vi "FGV_Timer.vi"(7 "Timer action (read)":T1=enum."Run") -> (3 "Numeric":dbl)   [LabVIEW 2020]
uses:
  #typedef_FGV_TimerAction_ex_4.ctl
panel:
  out "Time Elapsed?":bool
  in  "TimeToElapse (s)":dbl=10.0
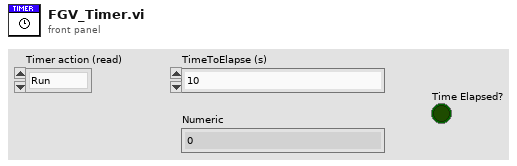
[diagram p1: front panel]
types:
  T1 = typedef "#typedef_FGV_TimerAction_ex_4.ctl" = enum16{"Reset", "Run", "Pause"}
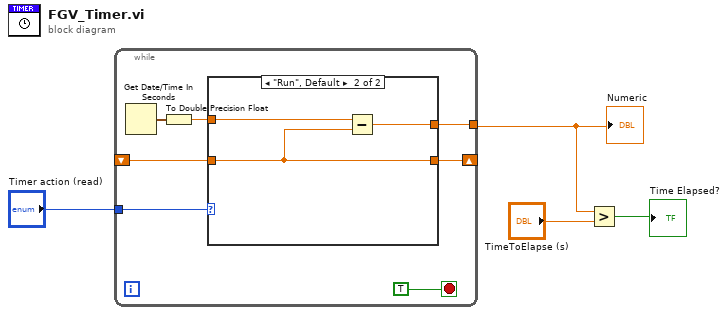
[diagram p0: block diagram]
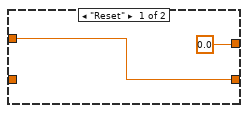
[diagram p2: hidden frame]
diagram:
  n1 = while {
    tunnel: "Timer action (read)" -> [w11]
    shift-right: [w8] -> _
    shift-left: _ -> [w6]
    tunnel: [w5] -> w3
    stop <- TRUE stop-if-true
    n2 = Get Date/Time In Seconds() -> (seconds since 1Jan1904=w9:timestamp)
    n3 = To Double Precision Float(number=w9) -> (double precision float=w7:dbl)
    n4 = case shown="\"Run\", Default" w11 {
      tunnel: [w13 w14] -> w8
      tunnel: w7 -> [w13 w16]
      tunnel: w6 -> [_ w14]
      tunnel: [0.0 w15] -> w5
      frame "Reset" {
      }
      frame "Run", Default {
        n5 = Subtract(x=w16, y=w14) -> (x-y=w15:dbl)
      }
    }
  }
  "Numeric" <- w3
  n6 = Greater?(x=w3, y="TimeToElapse (s)") -> (0:→"Time Elapsed?":bool)
